vi "Run.vi"(8 "error in (no error)":errorcluster, 11 "Telemetry in":refnum<class "Telemetry.lvclass">) -> (0 "error out":errorcluster, 3 "Telemetry out":refnum<class "Telemetry.lvclass">)   [LabVIEW 2018, in "Telemetry.lvclass"]
uses:
  Telemetry.lvclass
  Telemetry.lvclass/Telemetry.ctl
  Device/Device.lvclass
  StateMachine/State Machine.lvclass
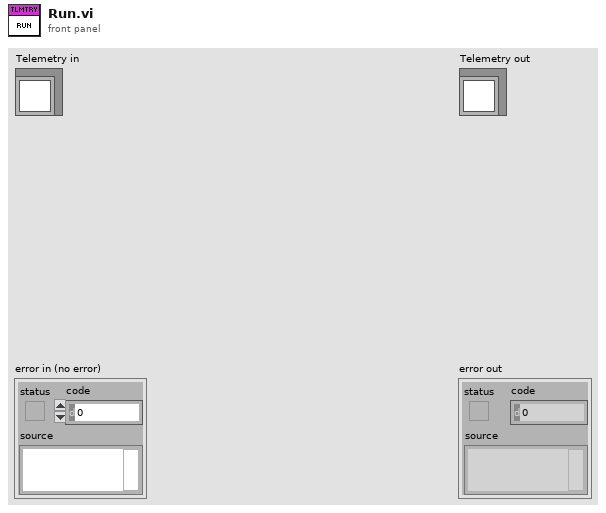
[diagram p1: front panel]
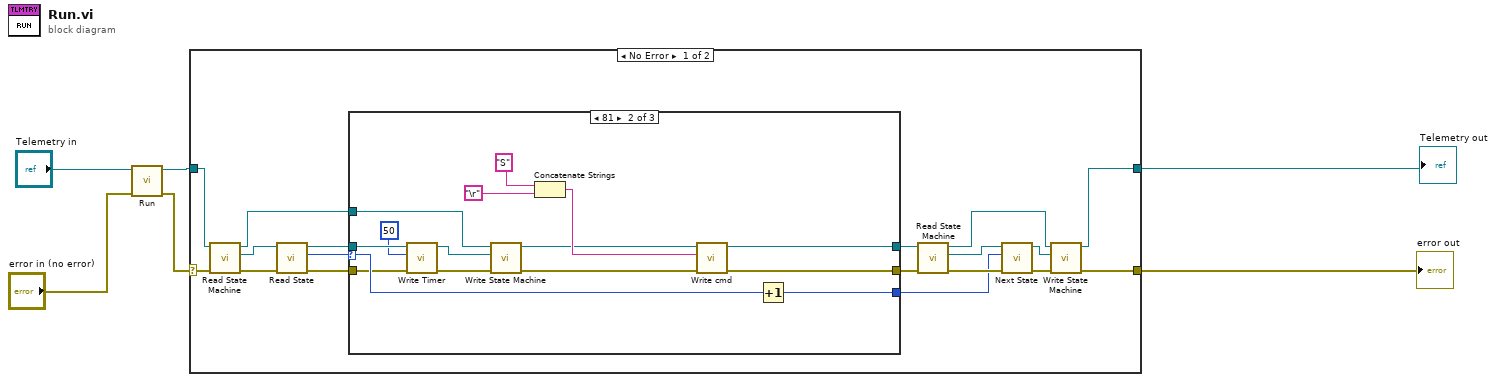
[diagram p0: block diagram]
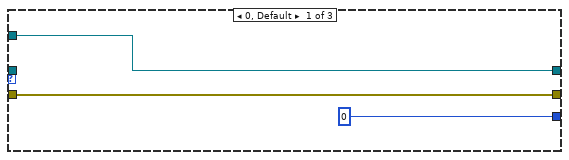
[diagram p2: hidden frame]
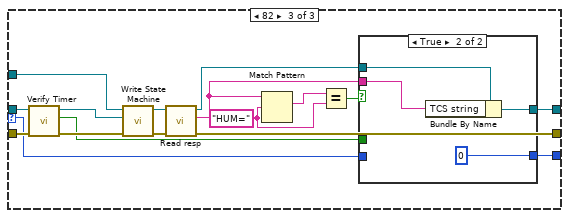
[diagram p3: hidden frame]
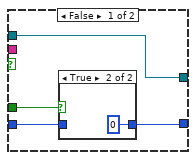
[diagram p4: hidden frame]
diagram:
  n1 = call-parent "Run.vi"("error in (no error)"="error in (no error)", "Device in"="Telemetry in") -> ("error out"=w3:errorcluster, "Device out"=w4:refnum<class "Telemetry.lvclass">)  [unwired: 8 in]
  n2 = case shown="No Error" w3 {
    selector: w3 -> [w23 w71]
    tunnel: [w15 w71] -> w1
    tunnel: w4 -> [w24 w70]
    tunnel: [w14 w70] -> w2
    frame No Error {
      n3 = call-dynamic "Read State Machine.vi"("error in (no error)"=w23, "Device in"=w24) -> ("error out"=w21:errorcluster, "State Machine.lvclass"=w22:refnum<class "State Machine.lvclass">, "Device out"=w12:refnum<class "Telemetry.lvclass">)  [unwired: 7 in]
      n4 = call-dynamic "Read State.vi"("error in (no error)"=w21, "State Machine in"=w22) -> ("error out"=w11:errorcluster, "State"=w13:i32, "State Machine out"=w7:refnum<class "State Machine.lvclass">)  [unwired: 7 in]
      n5 = case shown="81" w13 {
        selector: w13 -> [_ w42 w48]
        tunnel: w12 -> [w26 w33 w53]
        tunnel: w11 -> [w25 w31 w51]
        tunnel: [w25 w36 w57] -> w10
        tunnel: [w26 w37 w58] -> w9
        tunnel: [0 ("State") w41 w56] -> w8
        tunnel: w7 -> [_ w35 w55]
        frame 0, Default {
        }
        frame 81 {
          n6 = call-dynamic "Write Timer.vi"("error in (no error)"=w31, "Timer"=u32 50, "State Machine in"=w35) -> ("error out"=w30:errorcluster, "State Machine out"=w29:refnum<class "State Machine.lvclass">)  [unwired: 7 in]
          n7 = call-dynamic "Write State Machine.vi"("error in (no error)"=w30, "State Machine.lvclass"=w29, "Device in"=w33) -> ("error out"=w28:errorcluster, "Device out"=w32:refnum<class "Telemetry.lvclass">)  [unwired: 7 in]
          n8 = Concatenate Strings("S" ("cmd"), "\r") -> (w38:string)
          n9 = call-dynamic "Write cmd.vi"("error in (no error)"=w28, "cmd"=w38, "Device in"=w32) -> ("error out"=w36:errorcluster, "Device out"=w37:refnum<class "Telemetry.lvclass">)  [unwired: 7 in]
          n10 = Increment(x=w42) -> (x+1=w41:i32)
        }
        frame 82 {
          w45 = "HUM=" ("regular expression")
          n11 = call "Verify Timer.vi"("error in (no error)"=w51, "State Machine in"=w55) -> ("error out"=w52:errorcluster, "timeout"=w43:bool, "State Machine out"=w54:refnum<class "State Machine.lvclass">)  [unwired: 7 in]
          n12 = call-dynamic "Write State Machine.vi"("error in (no error)"=w52, "State Machine.lvclass"=w54, "Device in"=w53) -> ("error out"=w49:errorcluster, "Device out"=w50:refnum<class "Telemetry.lvclass">)  [unwired: 7 in]
          n13 = call-dynamic "Read resp.vi"("error in (no error)"=w49, "Device in"=w50) -> ("error out"=w57:errorcluster, "resp"=w44:string, "Device out"=w59:refnum<class "Telemetry.lvclass">)  [unwired: 7 in]
          n14 = Match Pattern(string=w44, regular expression=w45) -> (match substring=w46:string)  [unwired: 1 in, 3 out]
          n15 = Equal?(x=w46, y=w45) -> (x = y?=w47:bool)
          n16 = case shown="True" w47 {
            tunnel: w59 -> [w63 w69]
            tunnel: [w63 w68] -> w58
            tunnel: [w61 0] -> w56
            tunnel: w48 -> [w62 _]
            tunnel: w44 -> [_ w66]
            tunnel: w43 -> [w60 _]
            frame False {
              n17 = case shown="True" w60 {
                tunnel: w62 -> [w64 _]
                tunnel: [w64 0 ("State")] -> w61
                frame False {
                }
                frame True {
                }
              }
            }
            frame True {
              n18 = Bundle By Name(cluster=w69, "TCS string"=w66) -> (w68:refnum<class "Telemetry.lvclass">)
            }
          }
        }
      }
      n19 = call-dynamic "Read State Machine.vi"("error in (no error)"=w10, "Device in"=w9) -> ("error out"=w17:errorcluster, "State Machine.lvclass"=w19:refnum<class "State Machine.lvclass">, "Device out"=w18:refnum<class "Telemetry.lvclass">)  [unwired: 7 in]
      n20 = call "Next State.vi"("error in (no error)"=w17, "New_State"=w8, "State Machine in"=w19) -> ("error out"=w16:errorcluster, "State Machine out"=w20:refnum<class "State Machine.lvclass">)  [unwired: 7 in]
      n21 = call-dynamic "Write State Machine.vi"("error in (no error)"=w16, "State Machine.lvclass"=w20, "Device in"=w18) -> ("error out"=w15:errorcluster, "Device out"=w14:refnum<class "Telemetry.lvclass">)  [unwired: 7 in]
    }
    frame Error {
    }
  }
  "error out" <- w1
  "Telemetry out" <- w2
